vi "OpenCameraComms.vi"(8 "error in (no error)":errorcluster, 9 "Camera Occurance":refnum<k4>, 11 "SerialPortRef":T1) -> (0 "error out":errorcluster, 3 "SerialRefOut":T1)   [LabVIEW 2017, in "VisionHW.lvlib"]
uses:
  VisionHW.lvlib
  <vilib>/Rock Robotics/WPI/SerialPort/WPI_SerialPortRef.ctl
  <vilib>/Rock Robotics/WPI/SerialPort/WPI_SerialPort.ctl
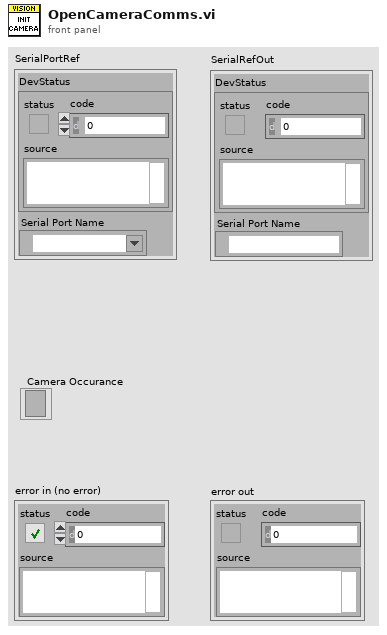
[diagram p1: front panel]
types:
  T1 = typedef "WPI_SerialPortRef.ctl" = cluster{"DevStatus":errorcluster, "Serial Port Name":refnum<visa-resource-name>}
  T2 = typedef "WPI_SerialPort.ctl" = enum16{"Onboard RS-232", "MXP TTL", "USB 1", "USB 2"}
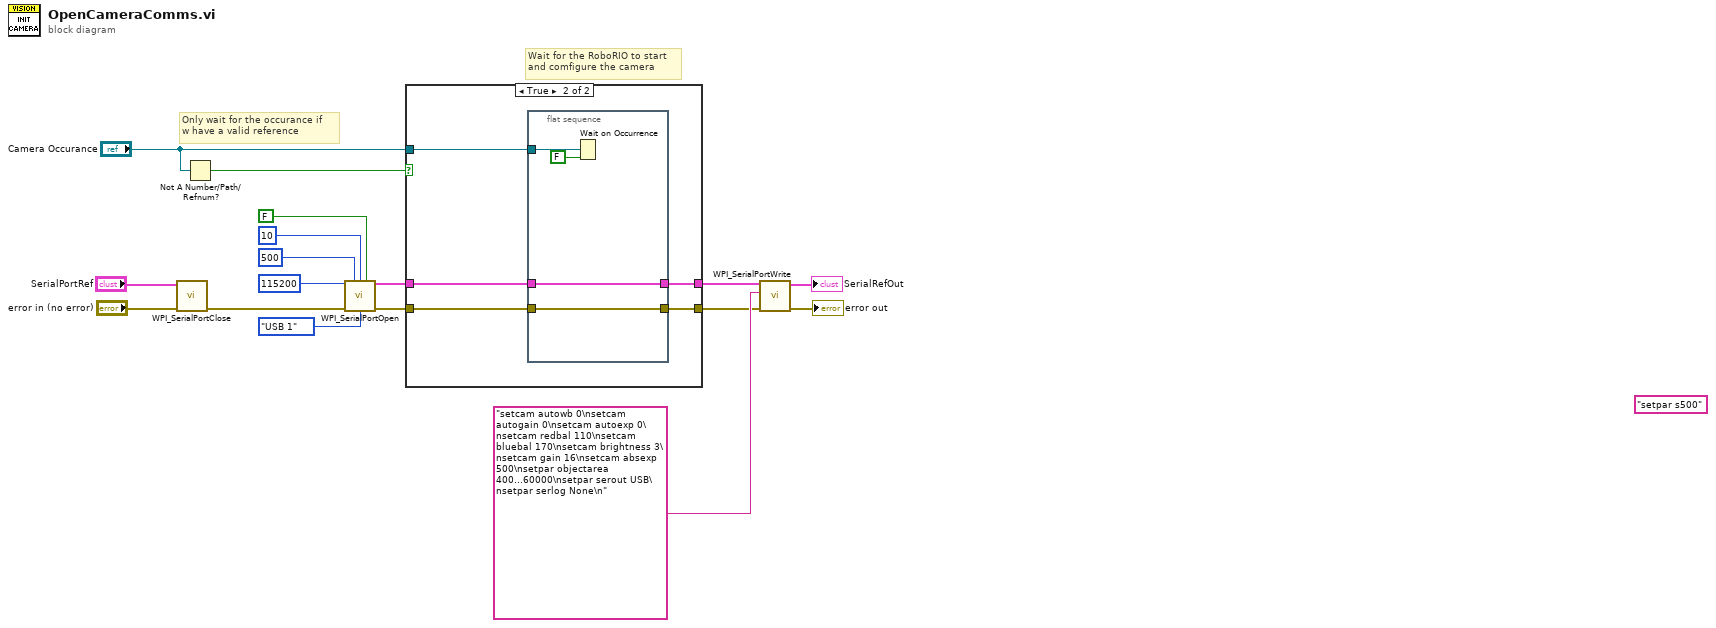
[diagram p0: block diagram]
diagram:
  (unwired) "setpar s500" ("write buffer")
  # "Only wait for the occurance if\nw have a valid reference"
  # "Wait for the RoboRIO to start\nand comfigure the camera"
  n1 = call <vilib>:"WPI_SerialPortClose.vi"("error in (no error)"="error in (no error)", "SerialPortRef"="SerialPortRef") -> ("error out"=w3:errorcluster)  [unwired: 9 in]
  n2 = Not A Number/Path/Refnum?(number/path/refnum="Camera Occurance") -> (NaN/Path/Refnum?=w2:bool)
  n3 = call <vilib>:"WPI_SerialPortOpen.vi"("Baud Rate"=u32 115200, "Timeout Value (ms)"=u32 500, "Termination Char (0xA = '\\n' = LF)"=u8 10 ("Termination Char (0xA = '\\n' = LF)"), "Enable Termination Char? (T)"=FALSE, "error in (no error)"=w3, "Serial Port"=WPI_SerialPort."USB 1") -> ("SerialPortRef"=w9:T1, "error out"=w8:errorcluster)  [unwired: 8 in]
  n4 = case shown="True" w2 {
    tunnel: w9 -> [w19 w24]
    tunnel: w8 -> [w18 w23]
    tunnel: [w19 w22] -> w7
    tunnel: [w18 w21] -> w6
    tunnel: "Camera Occurance" -> [_ w20]
    frame False {
    }
    frame True {
      n5 = flat-sequence {
        tunnel: w24 -> [w27]
        tunnel: w23 -> [w28]
        tunnel: [w27] -> w22
        tunnel: [w28] -> w21
        tunnel: w20 -> [w25]
        frame #0 {
          n6 = Wait on Occurrence(1:FALSE ("ignore previous (T)"), 2:w25) -> ()  [unwired: 1 in, 1 out]
        }
      }
    }
  }
  n7 = call <vilib>:"WPI_SerialPortWrite.vi"("error in (no error)"=w6, "Buffer"="setcam autowb 0\nsetcam autogain 0\nsetcam autoexp 0\nsetcam redbal 110\nsetcam bluebal 170\nsetcam brightness 3\nsetcam gain 16\nsetcam absexp 500\nsetpar objectarea 400...60000\nsetpar serout USB\nsetpar serlog None\n" ("write buffer"), "SerialPortRef"=w7) -> ("error out"=→"error out":errorcluster, "SerialPortRef"=→"SerialRefOut":T1)  [unwired: 6 in, 1 out]
